vi "PF_Conversion.vi"(0 "Intensity":dbl[](array[numeric]), 1 "xFit":sgl[](array[numeric]), 2 "yFit":dbl[](array[numeric])) -> (7 "Phase":cluster{"Ramp Pattern":dbl[], "phase out":dbl[]}(graph))   [LabVIEW 2020]
uses:
  <vilib>/Analysis/1siggen.llb/Ramp Pattern by Delta.vi
  <vilib>/Analysis/NI_AALBase.lvlib
panel:
  out "Phase Array":dbl[](array[numeric]) format="%.2f"
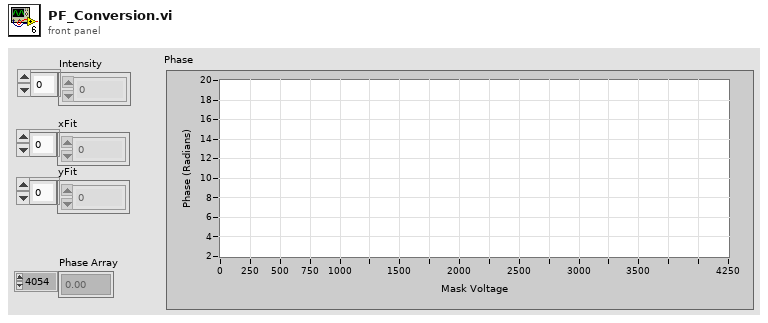
[diagram p1: front panel]
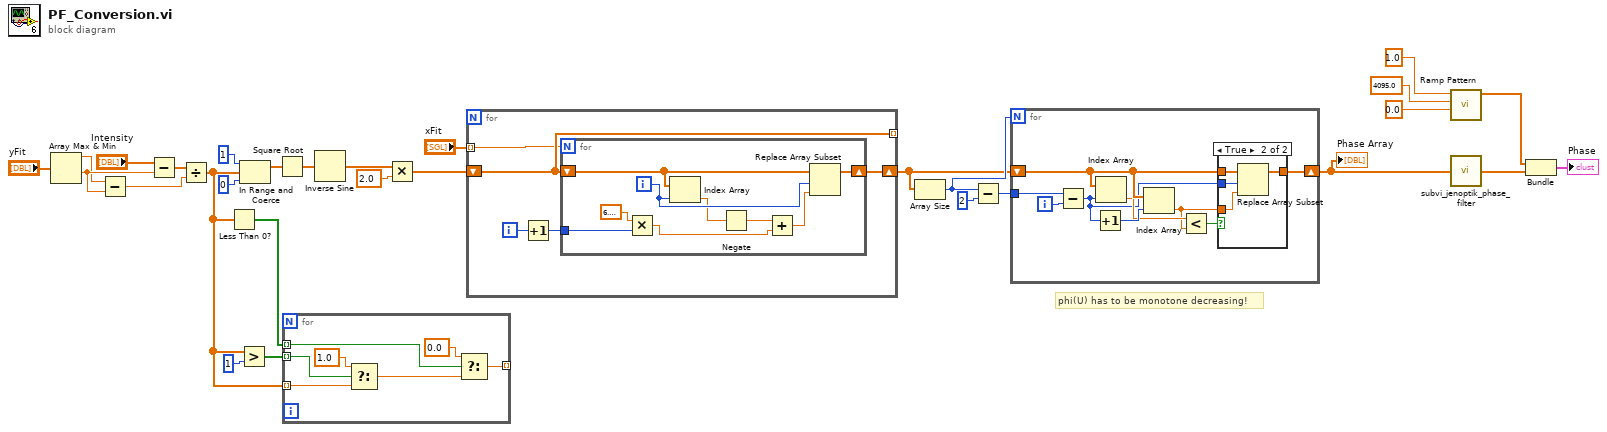
[diagram p0: block diagram]
diagram:
  # "phi(U) has to be monotone decreasing!"
  n1 = Array Max & Min(array="yFit") -> (max value=w20:dbl, min value=w21:dbl)  [unwired: 2 out]
  n2 = Subtract(x=w20, y=w21) -> (x-y=w23:dbl)
  n3 = Subtract(x="Intensity", y=w21) -> (x-y=w22:dbl[])
  n4 = Divide(x=w22, y=w23) -> (x/y=w18:dbl[])
  n5 = Less Than 0?(x=w18) -> (x < 0?=w26:bool[])
  n6 = Greater?(x=w18, y=1) -> (0:w25:bool[])
  n7 = In Range and Coerce(upper limit=1, x=w18, lower limit=0) -> (coerced(x)=w15:dbl[])  [unwired: 1 out]
  n8 = Square Root(x=w15) -> (sqrt(x)=w27:dbl[])
  n9 = for {
    tunnel: w25 -> [w36] mode=indexing
    tunnel: w18 -> [w34] mode=indexing
    tunnel: w26 -> [w32] mode=indexing
    tunnel: [w30] -> _ mode=indexing
    n10 = Select(t=1.0, s=w36, f=w34) -> (s? t:f=w33:dbl)
    n11 = Select(t=0.0, s=w32, f=w33) -> (s? t:f=w30:dbl)
  }
  n12 = Inverse Sine(1:w27) -> (0:w28:dbl[])
  n13 = Multiply(x=w28, y=2.0 ("t")) -> (x*y=w19:dbl[])
  n14 = for {
    shift-right: [w41] -> w2
    shift-left: w19 -> [w40]
    tunnel: [w40] -> _ mode=indexing
    tunnel: "xFit" -> [w37] mode=indexing
    i -> [w39]
    n15 = Increment(x=w39) -> (x+1=w38:i32)
    n16 = for {
      N: w37 -> [_]
      shift-right: [w48] -> w41
      shift-left: w40 -> [w49]
      tunnel: w38 -> [w43]
      i -> [w50]
      n17 = Multiply(x=6.283185307179586, y=w43) -> (x*y=w42:dbl)
      n18 = Index Array(array=w49, index=w50) -> (element=w47:dbl)
      n19 = Negate(x=w47) -> (-x=w46:dbl)
      n20 = Add(x=w46, y=w42) -> (x+y=w45:dbl)
      n21 = Replace Array Subset(array=w49, new element=w45, index=w50) -> (w48:dbl[])
    }
  }
  n22 = Array Size(array=w2) -> (size(s)=w5:i32)
  n23 = Subtract(x=w5, y=2) -> (x-y=w4:i32)
  n24 = for {
    N: w5 -> [_]
    shift-right: [w59] -> w1
    shift-left: w2 -> [w55]
    tunnel: w4 -> [w58]
    i -> [w57]
    n25 = Subtract(x=w58, y=w57) -> (x-y=w51:i32)
    n26 = Increment(x=w51) -> (x+1=w56:i32)
    n27 = Index Array(array=w55, index=w51) -> (element=w54:dbl)
    n28 = Index Array(array=w55, index=w56) -> (element=w52:dbl)
    n29 = Less?(x=w54, y=w52) -> (x < y?=w53:bool)
    n30 = case shown="True" w53 {
      tunnel: [w60 w64] -> w59
      tunnel: w55 -> [w60 w63]
      tunnel: w52 -> [_ w62]
      tunnel: w51 -> [_ w61]
      frame False {
      }
      frame True {
        n31 = Replace Array Subset(array=w63, new element=w62, index=w61) -> (w64:dbl[])
      }
    }
  }
  "Phase Array" <- w1
  n32 = call-poly <vilib>:"Ramp Pattern.vi"("start"=0.0, "end"=4095.0, "delta"=1.0) -> ("Ramp Pattern"=w10:dbl[])  [unwired: 6 in, 2 out]
  n33 = call "subvi_jenoptik_phase_filter.vi"("phase in"=w1) -> ("phase out"=w9:dbl[])  [unwired: 13 in, 1 out]
  n34 = Bundle("Ramp Pattern"=w10, "phase out"=w9) -> (→"Phase":cluster{"Ramp Pattern":dbl[], "phase out":dbl[]})  [unwired: 1 in]
